vi "Accumulate Execution Time.vi"(7 "Method Name":string, 9 "Execution Time":dbl, 11 "Test Result Tree V2 in":refnum<class "Test Result Tree V2.lvclass">) -> (3 "Test Result Tree V2 out":refnum<class "Test Result Tree V2.lvclass">)   [LabVIEW 2020, in "Test Result Tree V2.lvclass"]
uses:
  Test Result Tree V2.lvclass
  Test Result Tree V2.lvclass/Test Result Tree V2.ctl
  <vilib>/Utility/miscctls.llb/LVMapReplaceAction.ctl
  Utilities/LUnit Utilities.lvlib
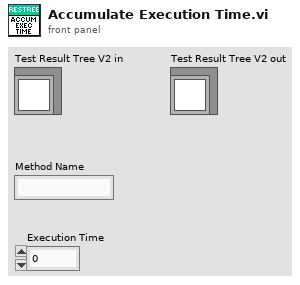
[diagram p1: front panel]
types:
  T1 = typedef "LVMapReplaceAction.ctl" = enum32{"Modify Entry only if found", "Add or Modify Entry", "Delete Entry"}
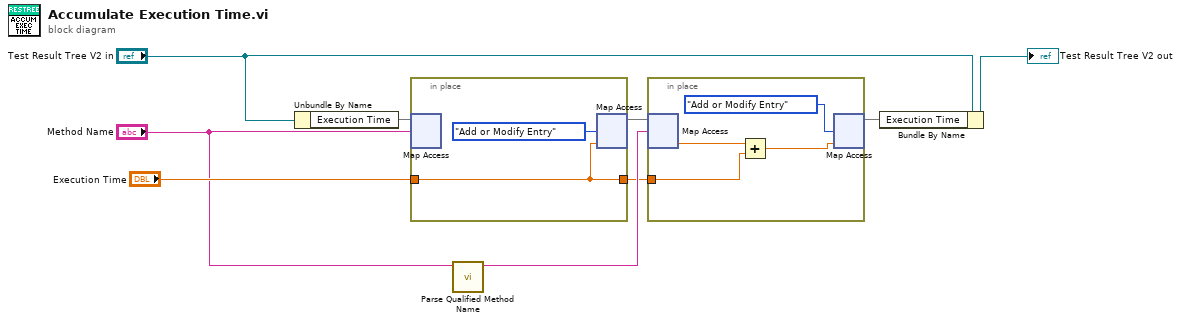
[diagram p0: block diagram]
diagram:
  n1 = Unbundle By Name("Test Result Tree V2 in") -> ("Execution Time"=w7:map{string, dbl})
  n2 = in-place {
    in-place-border: "Execution Time" -> [w10]
    in-place-border: [w10] -> w1
    n3 = in-place-map #1(w7, "Method Name") -> ()  [unwired: 1 in, 2 out]
    n4 = in-place-map #1(w10, LVMapReplaceAction."Add or Modify Entry" ("action")) -> (w4:map{string, dbl})  [unwired: 2 out]
  }
  n5 = call "Parse Qualified Method Name.vi"("Case"="Method Name") -> ("Test Case Class Name"=w2:string)  [unwired: 9 in, 1 out]
  n6 = in-place {
    in-place-border: w1 -> [w12]
    n7 = in-place-map #2(w4, w2) -> (w14:dbl)  [unwired: 1 in, 1 out]
    n8 = Add(x=w14, y=w12) -> (x+y=w13:dbl)
    n9 = in-place-map #2(w13, LVMapReplaceAction."Add or Modify Entry" ("action")) -> (w3:map{string, dbl})  [unwired: 2 out]
  }
  n10 = Bundle By Name(cluster="Test Result Tree V2 in", "Execution Time"=w3) -> (→"Test Result Tree V2 out":refnum<class "Test Result Tree V2.lvclass">)
